vi "Ball Carrying Logic.vi"(0 "Backwards Trigger":dbl, 1 "Fire from Load Delay":i32, 2 "Angle in":dbl, 5 "Boolean 2":bool, 7 "Rollers Active? in":bool, 9 "Safty Frist Angle":dbl, 12 "Intake Angle":dbl, 13 "Intake at Dangerous Height?":bool, 14 "Ball Loaded? in":bool) -> (4 "Rollers Active? out":bool, 6 "Angle out":dbl, 8 "f":dbl, 10 "Ball Loaded? out":bool)   [LabVIEW 2015]
uses:
  Common Code/Change Detect Boolean.vi
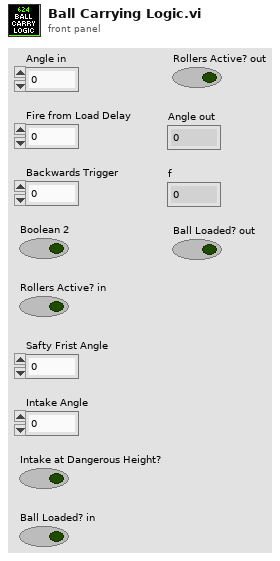
[diagram p1: front panel]
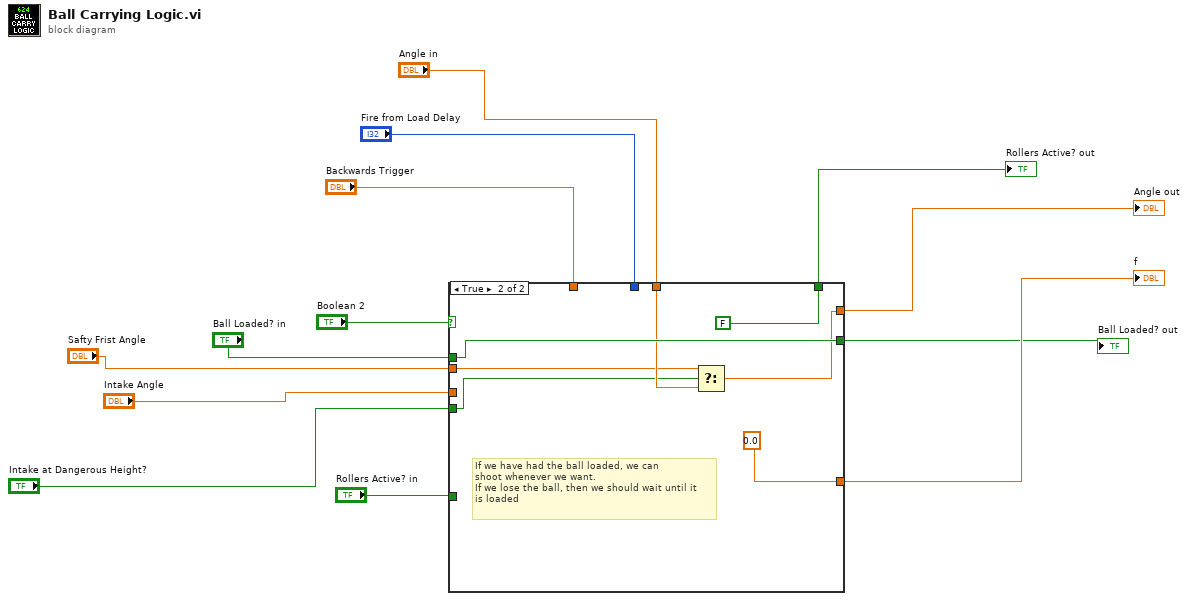
[diagram p0: block diagram]
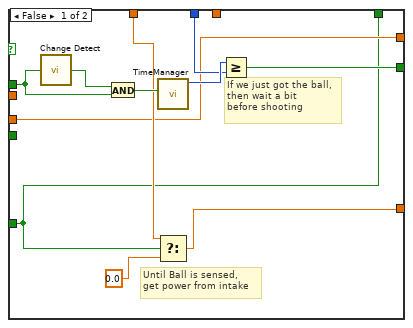
[diagram p2: hidden frame]
diagram:
  n1 = case shown="True" "Boolean 2" {
    tunnel: "Fire from Load Delay" -> [w21 _]
    tunnel: "Ball Loaded? in" -> [w20 w31]
    tunnel: [w19 w31] -> w1
    tunnel: [w17 0.0 ("f")] -> w7
    tunnel: "Rollers Active? in" -> [w14 _]
    tunnel: "Backwards Trigger" -> [w16 _]
    tunnel: [w14 FALSE] -> w6
    tunnel: "Angle in" -> [_ w28]
    tunnel: [w15 w25] -> w9
    tunnel: "Intake Angle" -> [w15 _]
    tunnel: "Intake at Dangerous Height?" -> [_ w27]
    tunnel: "Safty Frist Angle" -> [_ w26]
    frame False {
      # "Until Ball is sensed,\nget power from intake"
      # "If we just got the ball,\nthen wait a bit\nbefore shooting"
      n2 = call-poly "Change Detect.vi"("In"=w20) -> ("Changed?"=w24:bool)
      n3 = And(x=w24, y=w20) -> (x .and. y?=w23:bool)
      n4 = call "TimeManager.vi"("Reset?"=w23) -> ("Time Since Reset"=w22:u32)  [unwired: 9 in, 1 out]
      n5 = Select(t=w16, s=w14, f=0.0 ("t")) -> (s? t:f=w17:dbl)
      n6 = Greater Or Equal?(x=w22, y=w21) -> (x >= y?=w19:bool)
    }
    frame True {
      # "If we have had the ball loaded, we can\nshoot whenever we want.\nIf we lose the ball, then we should wait until it\nis loaded"
      n7 = Select(t=w26, s=w27, f=w28) -> (s? t:f=w25:dbl)
    }
  }
  "Angle out" <- w9
  "f" <- w7
  "Rollers Active? out" <- w6
  "Ball Loaded? out" <- w1
